vi "SetParam.vi"(8 "error in (no error)":errorcluster caption="entrée d'erreur (pas d'erreur)", 10 "fetch_20newsgroups":T1={"subset"="train", "categories"=["None"], "shuffle"=TRUE, "random_state"=42, "remove"=[], "download_if_missing"=TRUE, "Returns"="Data"} {"random_state" min=-1}, 11 "20newsgroups.lvclass":refnum<class "20newsgroups.lvclass">) -> (0 "error out":errorcluster caption="sortie d'erreur", 3 "20newsgroups.lvclass 2":refnum<class "20newsgroups.lvclass">)   [LabVIEW 2020, in "20newsgroups.lvclass"]
doc: "Set Parameters"
uses:
  20newsgroups.lvclass
  20newsgroups.lvclass/20newsgroups.ctl
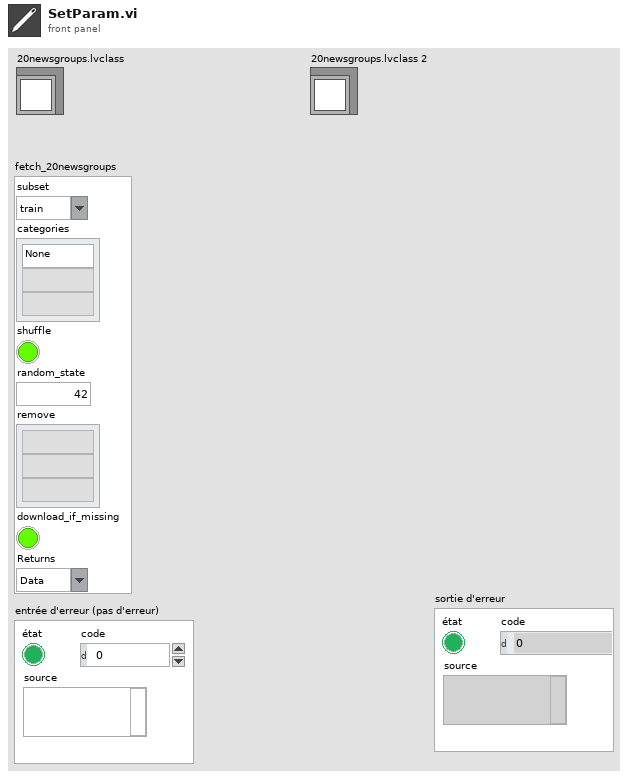
[diagram p1: front panel]
types:
  T1 = cluster{"subset":string, "categories":string[], "shuffle":bool, "random_state":i32, "remove":string[], "download_if_missing":bool, "Returns":string}
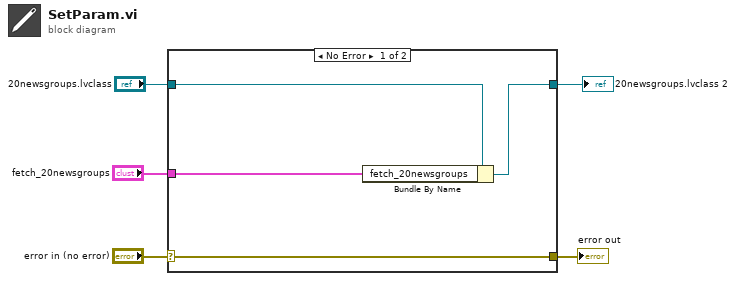
[diagram p0: block diagram]
diagram:
  n1 = case shown="No Error" "error in (no error)" {
    selector: "error in (no error)" -> [w9 w10]
    tunnel: [w9 w10] -> w4
    tunnel: [w7 w11] -> w2
    tunnel: "20newsgroups.lvclass" -> [w8 w11]
    tunnel: "fetch_20newsgroups" -> [w6 _]
    frame No Error {
      n2 = Bundle By Name(cluster=w8, "fetch_20newsgroups"=w6) -> (w7:refnum<class "20newsgroups.lvclass">)
    }
    frame Error {
    }
  }
  "error out" <- w4
  "20newsgroups.lvclass 2" <- w2
